vi "Position Backspace.vi"(8 "error in (no error)":errorcluster, 10 "Input field":refnum<vi>, 11 "Backspace":refnum<vi>) -> (0 "error out":errorcluster)   [LabVIEW 2014]
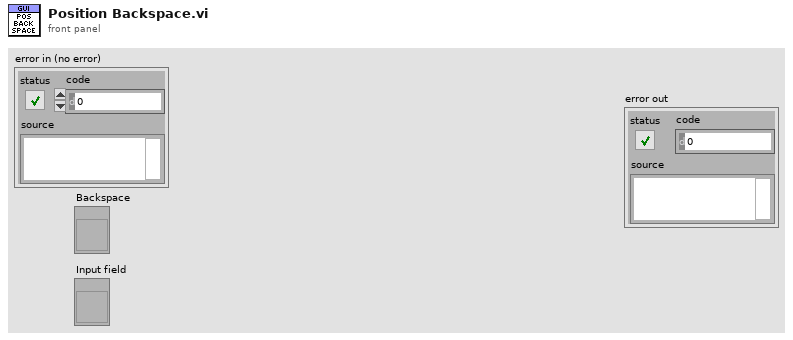
[diagram p1: front panel]
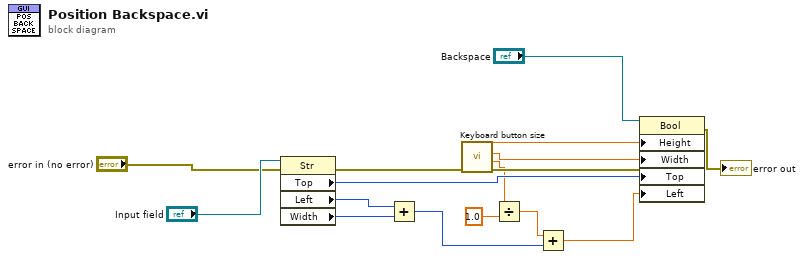
[diagram p0: block diagram]
diagram:
  n1 = property class="Str"(reference="Input field", error in="error in (no error)") -> (error out=w15:errorcluster, "Top"=w7:i32, "Left"=w9:i32, "Width"=w8:u32)  [unwired: 1 out]
  n2 = Add(x=w9, y=w8) -> (x+y=w3:u32)
  n3 = call "Keyboard button size.vi"("error in (no error)"=w15) -> ("error out"=w13:errorcluster, "Key Spacing"=w6:dbl, "Key Width"=w11:dbl, "Key Height"=w10:dbl)  [unwired: 7 in]
  n4 = Divide(x=w6, y=1.0) -> (x/y=w4:dbl)
  n5 = Add(x=w4, y=w3) -> (x+y=w2:dbl)
  n6 = property class="Bool"(reference="Backspace", error in=w13, "Height"=w10, "Width"=w11, "Top"=w7, "Left"=w2) -> (error out=→"error out":errorcluster)  [unwired: 1 out]
